vi "color-black.vi"(7 "url":string, 8 "error in (no error)":errorcluster, 11 "client handle":T1) -> (0 "error out":errorcluster, 3 "client handle out":T1)   [LabVIEW 2022 SP3]
uses:
  <vilib>/httpClient/ClientHandle.ctl
  <vilib>/httpClient/PUTBuffer.vi
  <vilib>/httpClient/LabVIEWHTTPClient.lvlib
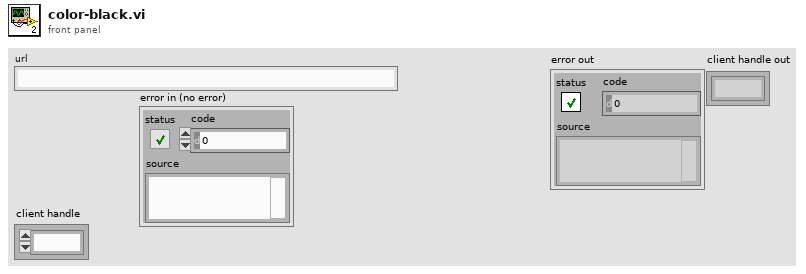
[diagram p1: front panel]
types:
  T1 = typedef "LabVIEWHTTPClient.lvlib/ClientHandle.ctl" = refnum<k1>
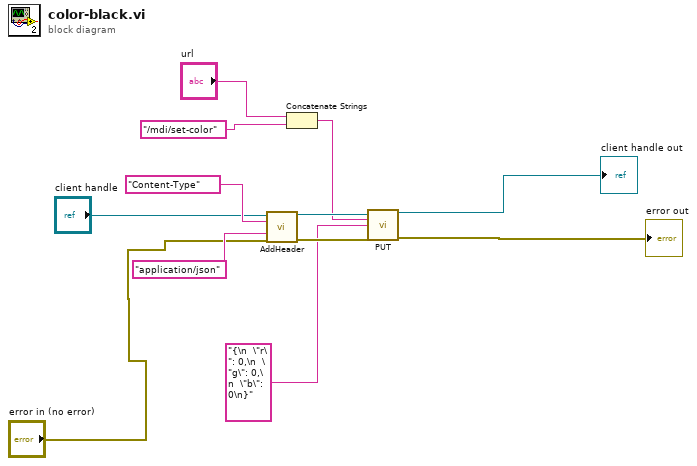
[diagram p0: block diagram]
diagram:
  n1 = call <vilib>:"AddHeader.vi"("client handle"="client handle", "header"="Content-Type", "value"="application/json", "error in (no error)"="error in (no error)") -> ("client handle out"=w11:T1, "error out"=w12:errorcluster)  [unwired: 10 in]
  n2 = Concatenate Strings("url", "/mdi/set-color" ("string")) -> (w5:string)
  n3 = call-poly <vilib>:"PUT.vi"("client handle"=w11, "url"=w5, "buffer"="{\n  \"r\": 0,\n  \"g\": 0,\n  \"b\": 0\n}", "error in (no error)"=w12) -> ("client handle out"=→"client handle out":T1, "error out"=→"error out":errorcluster)  [unwired: 8 in, 2 out]
